vi "Calibration.vi"(10 "Array 2":string[](array[string])=["192.168.10.20", "192.168.10.22"], 11 "SMA mode":bool=TRUE) -> (0 "error out":errorcluster)   [LabVIEW 2017]
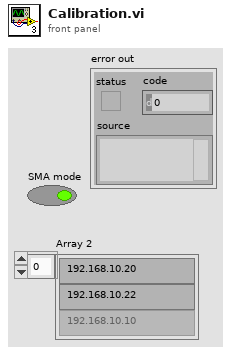
[diagram p1: front panel]
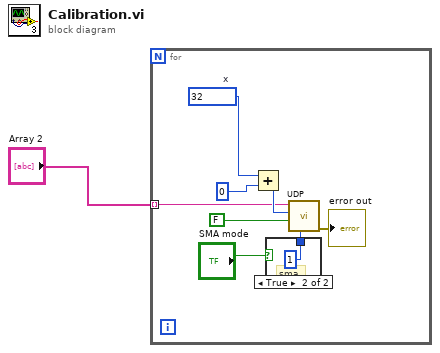
[diagram p0: block diagram]
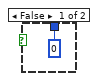
[diagram p2: hidden frame]
diagram:
  n1 = for {
    tunnel: "Array 2" -> [w3] mode=indexing
    w5 = u16 32  # x
    n2 = Add(x=w5, y=u32 0 ("Address")) -> (x+y=w4:u32)
    n3 = case shown="True" "SMA mode" {
      tunnel: [u8 0 ("In") u8 1 ("In")] -> w8
      frame False {
      }
      frame True {
        # "sma"
      }
    }
    n4 = call "UDP.vi"("In"=w8, "Read (TRUE)"=FALSE, "Address"=w4, "IP address"=w3) -> ("error out"=→"error out":errorcluster)  [unwired: 5 in, 1 out]
  }
